vi "Delete User Attribute.vi"(0 "User Configuration Manager in":refnum<class "User Configuration Manager.lvclass">, 5 "Username":string, 7 "Attribute Name":string, 11 "error in (no error)":errorcluster) -> (4 "User Configuration Manager out":refnum<class "User Configuration Manager.lvclass">, 6 "Found":bool, 15 "error out":errorcluster)   [LabVIEW 2019, in "User Configuration Manager.lvlib" / "User Configuration Manager.lvclass"]
doc: "Deletes the attrbute specifed by attribute name from the user specifiec by user name."
uses:
  <vilib>/gpm_packages/@cs/user-manager/Source/User Configuration Manager/User Configuration Manager.lvclass
  <vilib>/gpm_packages/@cs/user-manager/Source/User Configuration Manager/User Configuration Manager.lvclass/User Configuration Manager.ctl
  f4f2de71-e9cf-4401-ba7c-d1f782dd7fb6.vi
  <vilib>/gpm_packages/@cs/user-manager/Source/User Configuration Manager/Accessors/Read Linked List Ref .vi
  <vilib>/gpm_packages/@cs/linked-list/Source/Linked List/ILinkedList/ILinked List.lvclass
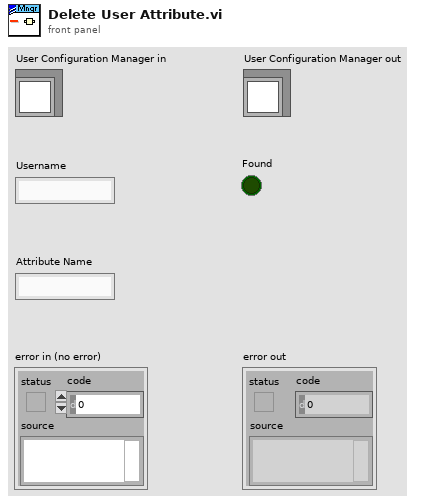
[diagram p1: front panel]
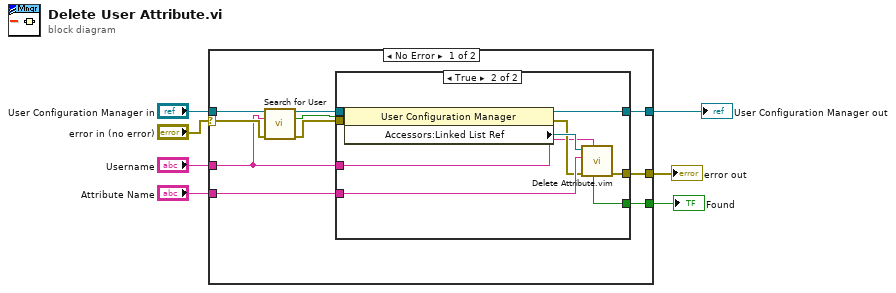
[diagram p0: block diagram]
diagram:
  n1 = case shown="No Error" "error in (no error)" {
    selector: "error in (no error)" -> [w10 w29]
    tunnel: "User Configuration Manager in" -> [w13 w30]
    tunnel: "Attribute Name" -> [w14 _]
    tunnel: "Username" -> [w9 _]
    tunnel: [w17 w30] -> w3
    tunnel: [w16 w29] -> w2
    tunnel: [w15 _] -> w1
    frame No Error {
      n2 = call-dynamic "Search for User.vi"("User Configuration Manager in"=w13, "Username"=w9, "error in (no error)"=w10) -> ("User Configuration Manager out"=w12:refnum<class "User Configuration Manager.lvclass">, "Found"=w8:bool, "error out"=w11:errorcluster)  [unwired: 10 in]
      n3 = case shown="True" w8 {
        tunnel: [w19 w28] -> w17
        tunnel: [w18 w26] -> w16
        tunnel: [_ w25] -> w15
        tunnel: w14 -> [_ w24]
        tunnel: w12 -> [w19 w22]
        tunnel: w11 -> [w18 w21]
        tunnel: w9 -> [_ w20]
        frame False {
        }
        frame True {
          n4 = property class="User Configuration Manager"(reference=w22, error in=w21) -> (reference out=w28:refnum<class "User Configuration Manager.lvclass">, error out=w23:errorcluster, "Accessors:Linked List Ref "=w27:refnum<data-value>)
          n5 = call "Delete Attribute.vim"("Linked List ID"=w20, "error in (no error)"=w23, "Attribute Name"=w24, "Linked List Ref"=w27) -> ("error out"=w26:errorcluster, "Found?"=w25:bool)  [unwired: 5 in, 1 out]
        }
      }
    }
    frame Error {
    }
  }
  "error out" <- w2
  "User Configuration Manager out" <- w3
  "Found" <- w1
